vi "8chanxyplot.vi"() -> ()   [LabVIEW 2013]
doc: "Cont(inuous) Acq(uire) & Chart (hw timed) demonstrates the hardware timed, non-buffered technique of data acquisition. The scan clock on the board controls acquisition timing. Acquired scans are read directly from the device's FIFO using AI Single Scan. \n\nThe acquisition is configured with no buffer, and the on-board scan clock started at the selected scan rate. In the first loop iteration, the newest (most recent) scan is read from the FIFO. In each subsequent loop iteration AI Single Scan is called to read the oldest scan from the FIFO. Then if a scan is missed because the acquisition does not keep up, an error message will be displayed, and the acquisition stopped. Each scan is plotted on the chart after it is read. \n\nA common reason to use non-buffered acquisition is that some kind of processing needs to be done for each data point. You will probably want to add more functions to the diagram to customize this VI for your application. The acquisition rate you can achieve depends on how much processing and display the VI must do. This VI calls a subVI named My Single-Scan Processing. Add whatever processing you need to this subVI, or replace it with one of your own. The data processing subVI also demonstrates how to use error clusters in your own subVIs, so they can be included in the error data flow chain.\n\nBefore running this VI, set the values of the controls on the front panel. Select Show Help Window from the Help menu to see a description of each control. If the values you select for all the controls are values you will usually use, select Make Current Values Default from the Operate menu and save the VI. Or, you may save individual control's default values by popping up on the control, selecting Data Operations, then selecting Make Current Value Default, and saving the VI."
uses:
  <vilib>/DAQmx/read.llb/DAQmx Read (Analog 2D DBL NChan NSamp).vi
  BiaxGlobals.vi
  <vilib>/DAQmx/create/channels.llb/DAQmx Create Channel (AI-Voltage-Basic).vi
  <vilib>/DAQmx/configure/timing.llb/DAQmx Timing (Sample Clock).vi
  Homegrown2/effectiveglobals.vi
  <vilib>/DAQmx/miscellaneous.llb/DAQmx Fill In Error Info.vi
panel:
  in  "Show plot":bool
  out "Zero Voltage Y":dbl
  in  "Calibration y-axis (V/unit)":dbl=0.0119 format="%#_6f"
  in  "Select y-axis":string(combo)="Shear load"
  in  "Calibration x-axis (V/unit)":dbl=1.5233 format="%#_6f"
  in  "Select x-axis":string(combo)="LP displacement"
  out "Offset Voltage 2":dbl=-4.85
  in  "Offset DCDT 2":bool
  out "Offset Voltage 1":dbl=-4.85
  in  "Offset DCDT 1":bool
  in  "Zero y-axis":bool
  in  "Reset plot":bool
  out "Zero Voltage X":dbl
  in  "Zero X-axis":bool
  out "Shear Load vs Displacement":cluster{"Y":dbl[], "Y":dbl[]}[](graph)
  out "element 11":string
  out "element 10":string
  out "element 9":string
  out "element 8":string
  out "element 7":string
  out "element 6":string
  out "element 5":string
  out "element 4":string
  out "element 3":string
  out "element 2":string
  out "element":string
  out "element":string
  out "Stress-strain-temp vs time (Voltage)":dbl[][](graph)
  out "Array 13":i32[][](array[numeric])
  out "Array 12":i32[][](array[numeric])
  out "AUX8 (ch11)":dbl format="%.4f"
  out "AUX7 (ch10)":dbl format="%.4f"
  out "Array 11":i32[][](array[numeric])
  out "Array 10":i32[][](array[numeric])
  out "AUX6 (ch9)":dbl format="%.4f"
  out "AUX5 (ch8)":dbl format="%.4f"
  out "Array 9":i32[][](array[numeric])
  out "Array 8":i32[][](array[numeric])
  out "Array 7":i32[][](array[numeric])
  out "Array 6":i32[][](array[numeric])
  out "Array 5":i32[][](array[numeric])
  out "Array 4":i32[][](array[numeric])
  out "Array 3":i32[][](array[numeric])
  out "Array 2":i32[][](array[numeric])
  out "Array":i32[][](array[numeric])
  out "AUX4 (ch7)":dbl format="%.4f"
  out "AUX3 (ch6)":dbl format="%.4f"
  out "AUX2 (ch5)":dbl format="%.4f"
  out "AUX1 (ch4)":dbl format="%.4f"
  out "10000":bool
  in  "10 kHz":bool
  out "Processor scan rate":i32
  out "Present sample number":i32
  in  "1 Hz":bool
  out "1":bool
  out "10":bool
  out "100":bool
  out "1000":bool
  in  "10 Hz":bool
  in  "100 Hz":bool
  in  "1000 Hz":bool
  out "Data Recording Rate":i32(slide) scale=1.0..10000.0
  out "Write interval":i32
  out "Write countdown":i32
  out "Time into data acq. (s)":i32
  out "Saved sample No.":i32
  out "Record rate (samp/s)":i32
  out "No. of scans in backlog":i32
  out "Vert LVDT (ch3)":dbl format="%.4f"
  out "Vert Load (ch2)":dbl format="%.4f"
  out "Hor Load (ch0)":dbl format="%.4f"
  out "Hor LVDT (ch1)":dbl format="%.4f"
  in  "stop":bool
  # "Input Signals (volts)"
  # "To File (32 bit)"
  # "S\nI\nG\nN\nA\nL\n\nV\nO\nL\nT\nA\nG\nE"
  # "Timestamp"
  # "Acquisition Statistics"
  # "Data Recording Info"
  # "Sample (point) Number"
  # "NOTE:  This instrument will write data (time channel then Channels 0-3) to a user defined filename.  The file is written in binary format without a header.  The time channel is comprised of numbers indicating the data recording frequency (eg 1, 10, 100, 1000, 10000  samples per second)."
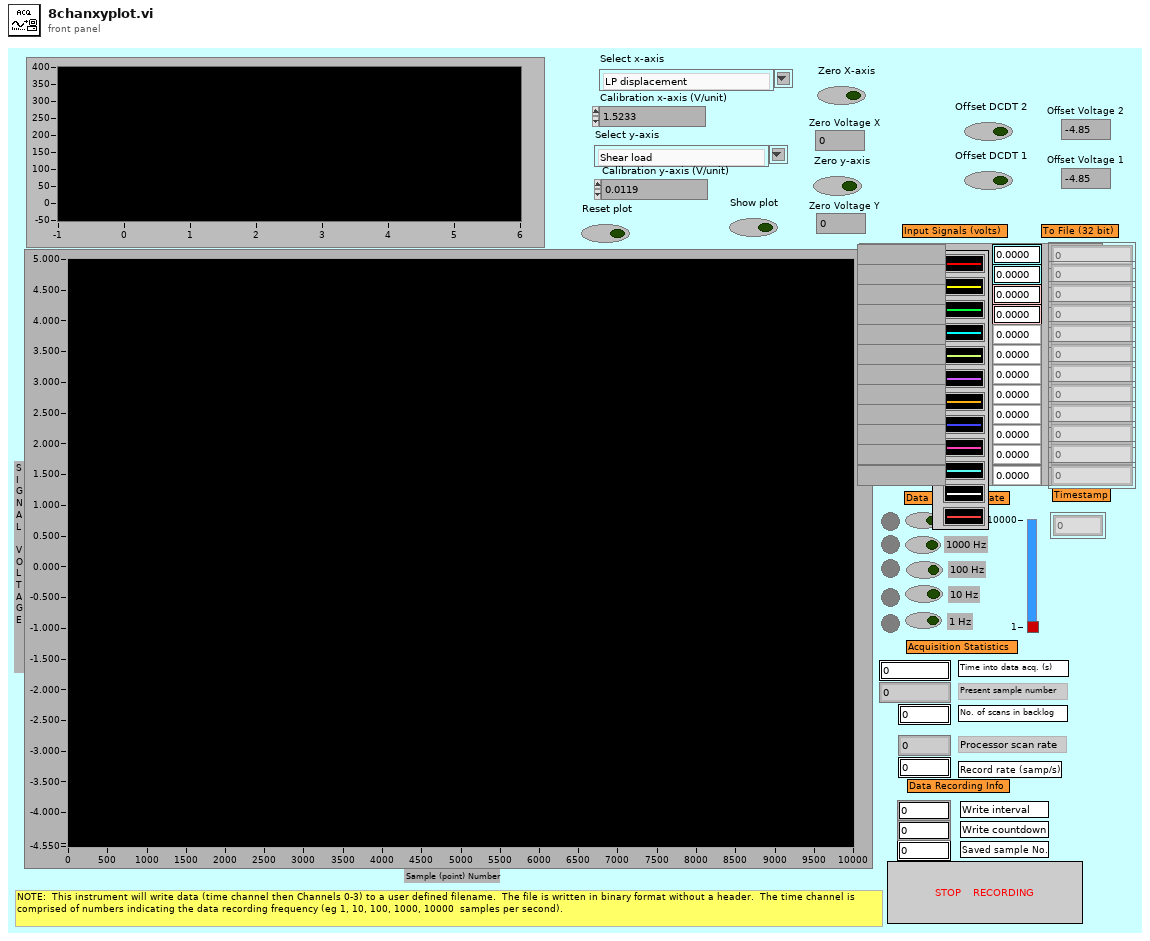
[diagram p1: front panel]
types:
  T1 = enum16{"big-endian, network order", "native, host order", "little-endian"}
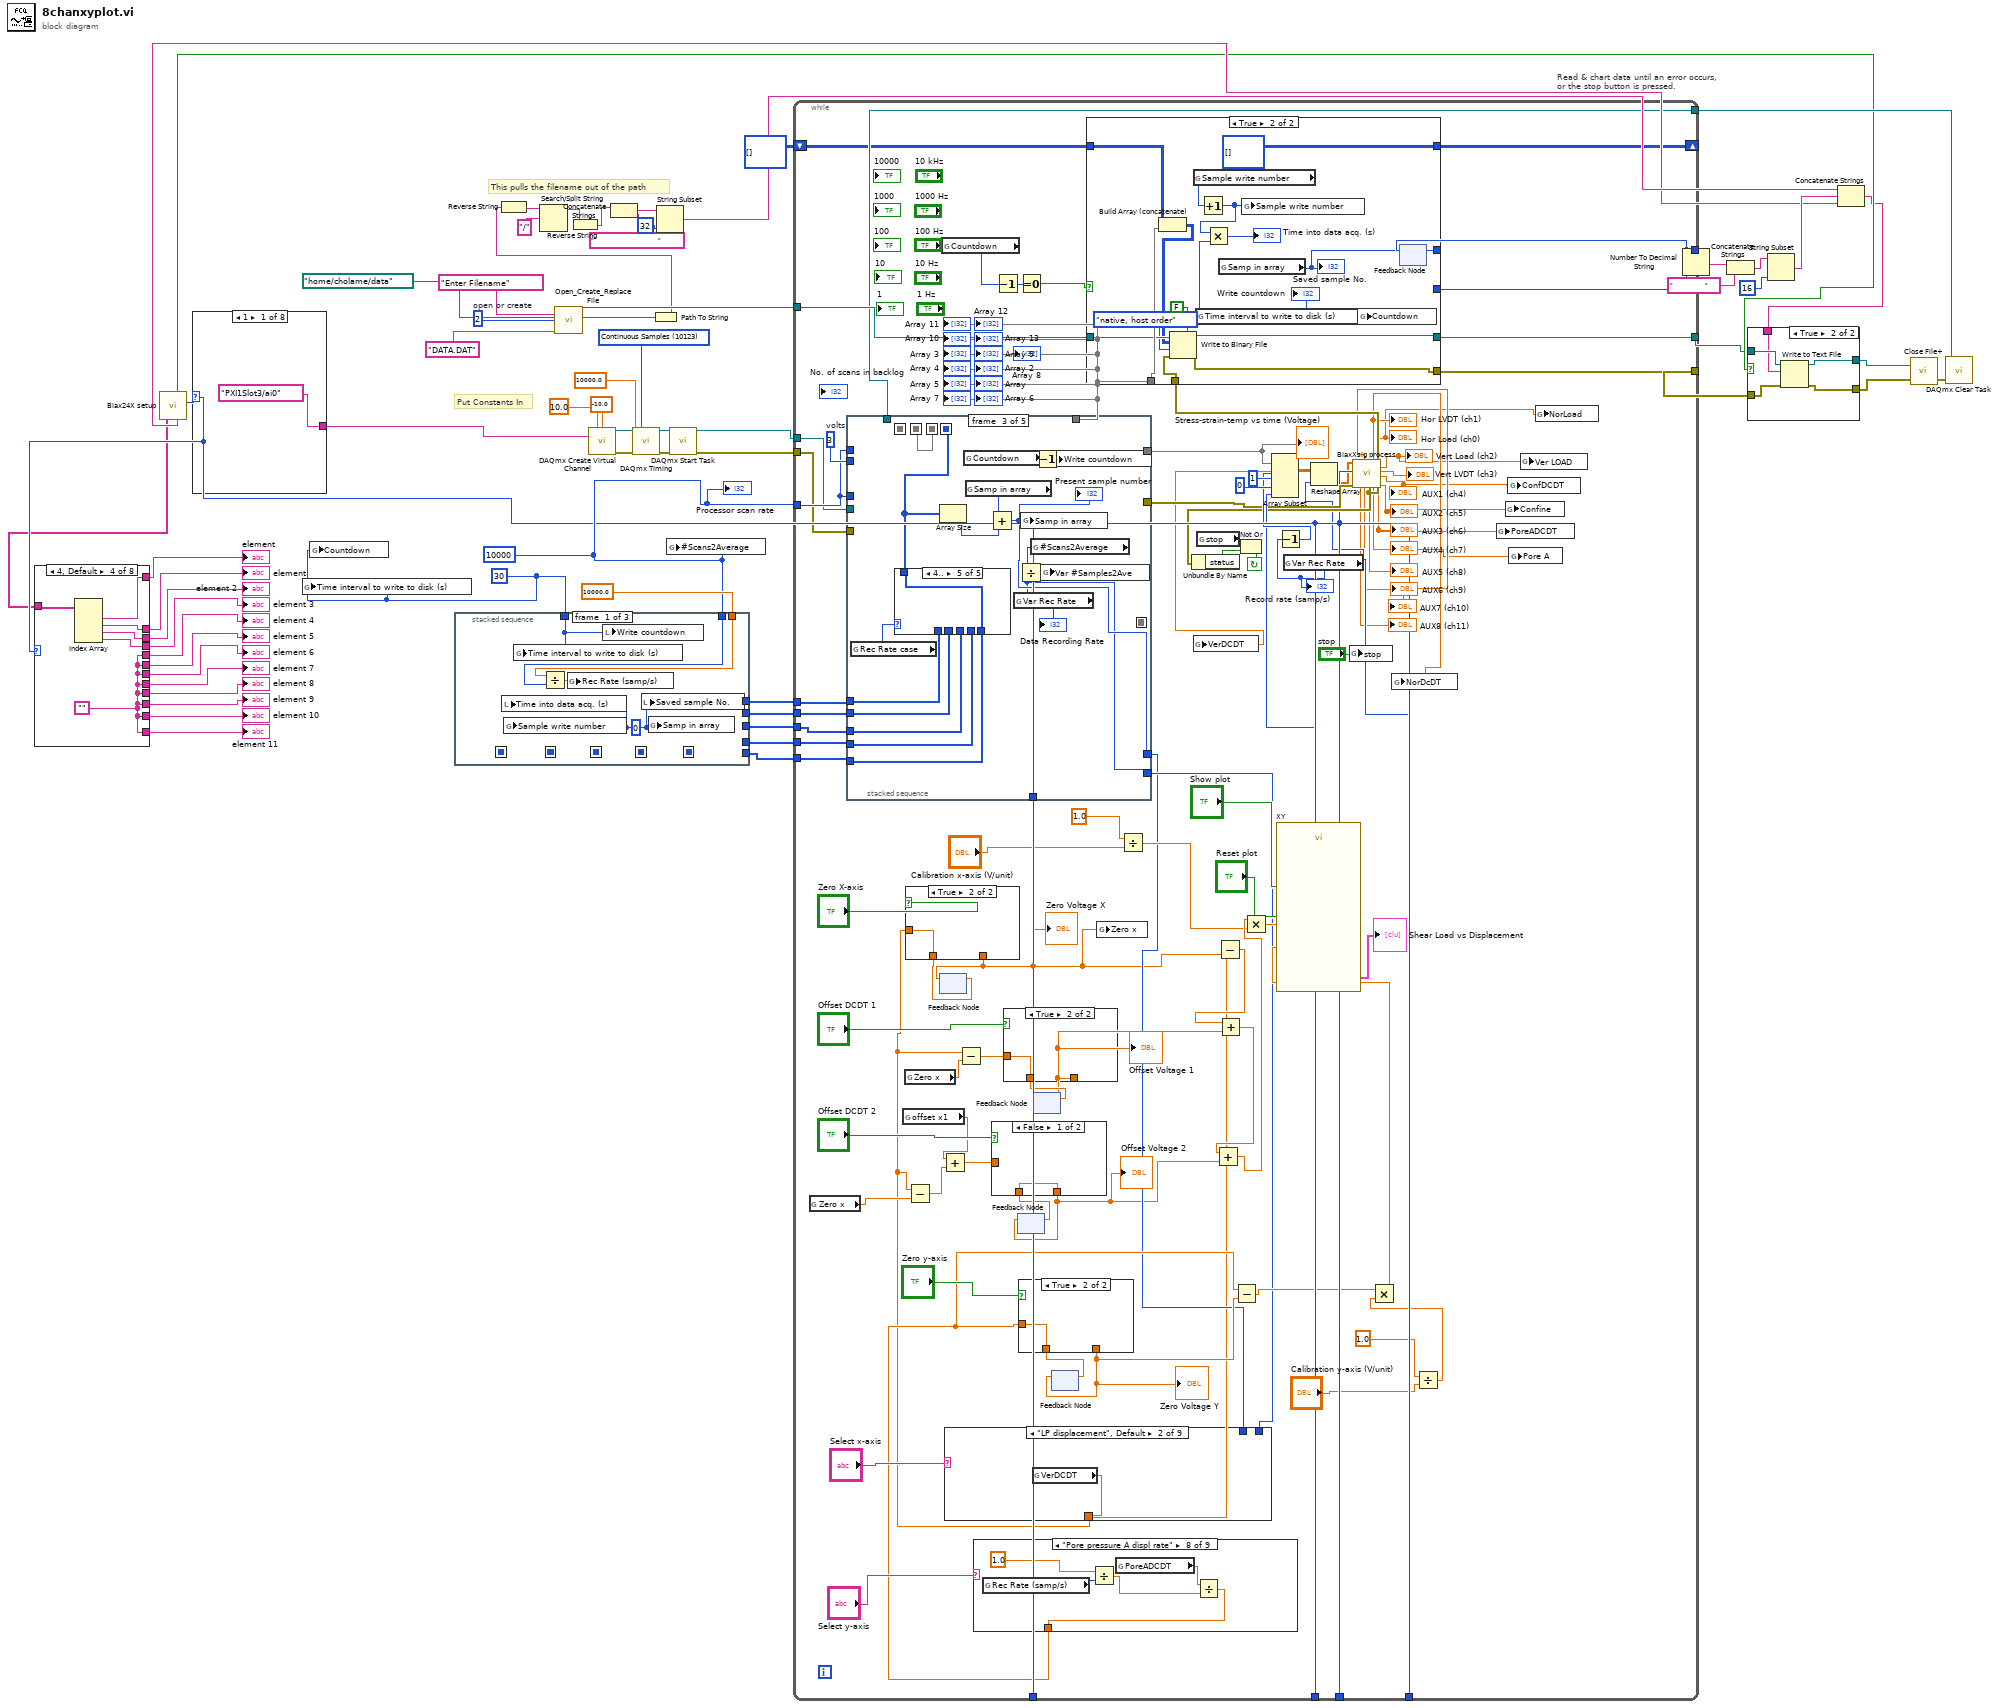
[diagram p0: block diagram]
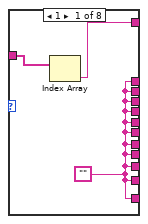
[diagram p2: hidden frame]
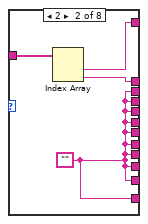
[diagram p3: hidden frame]
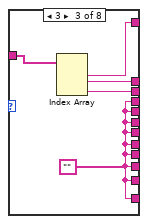
[diagram p4: hidden frame]
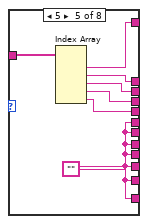
[diagram p5: hidden frame]
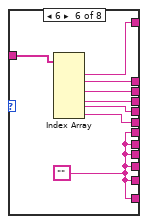
[diagram p6: hidden frame]
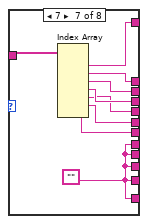
[diagram p7: hidden frame]
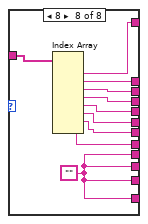
[diagram p8: hidden frame]
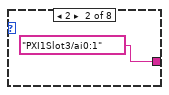
[diagram p10: hidden frame]
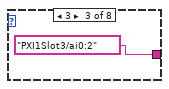
[diagram p11: hidden frame]
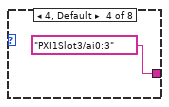
[diagram p12: hidden frame]
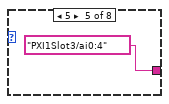
[diagram p13: hidden frame]
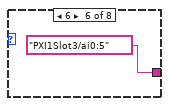
[diagram p14: hidden frame]
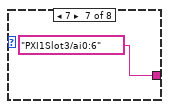
[diagram p15: hidden frame]
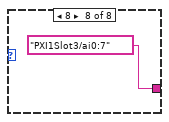
[diagram p16: hidden frame]
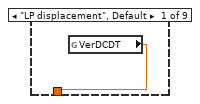
[diagram p17: hidden frame]
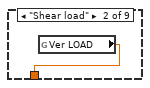
[diagram p18: hidden frame]
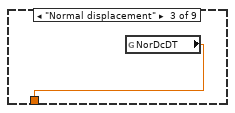
[diagram p19: hidden frame]
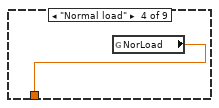
[diagram p20: hidden frame]
diagram:
  w34 = 10000 ("Number of scans")
  w33 = 30 ("Write time int (s)")
  w43 = 10123 items=["Finite Samples"=10178, "Continuous Samples"=10123, "Hardware Timed Single Point"=12522] ("sample mode")
  w64 = 2  # open or create
  # "This pulls the filename out of the path"
  # "Put Constants In"
  n1 = call "Biax24X setup.vi"() -> ("Footer String"=w22:string, "Number of Channels"=w15:i32, "ASCII footer 2"=w21:bool, "Channel Names"=w14:string[])  [unwired: 1 in, 4 out]
  n2 = case shown="4, Default" w15 {
    tunnel: w14 -> [w66 w70 w75 w81 w88 w96 w105 w116]
    tunnel: [w65 w71 w76 w82 w89 w97 w106 w115] -> w13
    tunnel: [w67 w69 w74 w80 w87 w95 w104 w114] -> w12
    tunnel: [w67 w68 w73 w79 w86 w94 w103 w113] -> w11
    tunnel: [w67 w68 w72 w78 w85 w93 w102 w112] -> w10
    tunnel: [w67 w68 w72 w77 w84 w92 w101 w111] -> w9
    tunnel: [w67 w68 w72 w77 w83 w91 w100 w110] -> w8
    tunnel: [w67 w68 w72 w77 w83 w90 w99 w109] -> w7
    tunnel: [w67 w68 w72 w77 w83 w90 w98 w108] -> w6
    tunnel: [w67 w68 w72 w77 w83 w90 w98 w107] -> w5
    tunnel: [w67 w68 w72 w77 w83 w90 w98 w107] -> w4
    tunnel: [w67 w68 w72 w77 w83 w90 w98 w107] -> w3
    tunnel: [w67 w68 w72 w77 w83 w90 w98 w107] -> w2
    frame 1 {
      w67 = ""
      n3 = Index Array(array=w66) -> (element=w65:string)  [unwired: 1 in]
    }
    frame 2 {
      w68 = ""
      n4 = Index Array(array=w70) -> (element #1=w71:string, element #2=w69:string)  [unwired: 2 in]
    }
    frame 3 {
      w72 = ""
      n5 = Index Array(array=w75) -> (element #1=w76:string, element #2=w74:string, element #3=w73:string)  [unwired: 3 in]
    }
    frame 4, Default {
      w77 = ""
      n6 = Index Array(array=w81) -> (element #1=w82:string, element #2=w80:string, element #3=w79:string, element #4=w78:string)  [unwired: 4 in]
    }
    frame 5 {
      w83 = ""
      n7 = Index Array(array=w88) -> (element #1=w89:string, element #2=w87:string, element #3=w86:string, element #4=w85:string, element #5=w84:string)  [unwired: 5 in]
    }
    frame 6 {
      w90 = ""
      n8 = Index Array(array=w96) -> (element #1=w97:string, element #2=w95:string, element #3=w94:string, element #4=w93:string, element #5=w92:string, element #6=w91:string)  [unwired: 6 in]
    }
    frame 7 {
      w98 = ""
      n9 = Index Array(array=w105) -> (element #1=w106:string, element #2=w104:string, element #3=w103:string, element #4=w102:string, element #5=w101:string, element #6=w100:string, element #7=w99:string)  [unwired: 7 in]
    }
    frame 8 {
      w107 = ""
      n10 = Index Array(array=w116) -> (element #1=w115:string, element #2=w114:string, element #3=w113:string, element #4=w112:string, element #5=w111:string, element #6=w110:string, element #7=w109:string, element #8=w108:string)  [unwired: 8 in]
    }
  }
  "element" <- w13
  "element" <- w12
  "element 2" <- w11
  "element 3" <- w10
  "element 4" <- w9
  "element 5" <- w8
  "element 6" <- w7
  "element 7" <- w6
  "element 8" <- w5
  "element 9" <- w4
  "element 10" <- w3
  "element 11" <- w2
  n11 = case shown="1" w15 {
    tunnel: [tag "PXI1Slot3/ai0" ("physical channels") tag "PXI1Slot3/ai0:1" ("physical channels") tag "PXI1Slot3/ai0:2" ("physical channels") tag "PXI1Slot3/ai0:3" ("physical channels") tag "PXI1Slot3/ai0:4" ("physical channels") tag "PXI1Slot3/ai0:5" ("physical channels") tag "PXI1Slot3/ai0:6" ("physical channels") tag "PXI1Slot3/ai0:7" ("physical channels")] -> w30
    frame 1 {
    }
    frame 2 {
    }
    frame 3 {
    }
    frame 4, Default {
    }
    frame 5 {
    }
    frame 6 {
    }
    frame 7 {
    }
    frame 8 {
    }
  }
  n12 = global write "BiaxGlobals.vi" "Time interval to write to disk (s)"(w33) -> ()
  n13 = global write "BiaxGlobals.vi" "Countdown"(w33) -> ()
  n14 = stacked-sequence {
    seq-local: [_ w145 _] -> [_ _ w158]
    seq-local: [_ w142 _] -> [_ _ w155]
    seq-local: [_ w137 _] -> [_ _ w157]
    seq-local: [_ w136 _] -> [_ _ w156]
    seq-local: [_ w131 _] -> [_ _ w154]
    tunnel: w33 -> [w125 _ _]
    tunnel: w34 -> [w129 _ _]
    tunnel: sgl 10000.0 ("actual scan rate") -> [w127 _ _]
    tunnel: [_ _ w158] -> w59
    tunnel: [_ _ w155] -> w58
    tunnel: [_ _ w157] -> w57
    tunnel: [_ _ w156] -> w56
    tunnel: [_ _ w154] -> w55
    frame #0 {
      w126 = i16 0
      n15 = local write "Time into data acq. (s)"(w126) -> ()
      n16 = global write "BiaxGlobals.vi" "Sample write number"(w126) -> ()
      n17 = global write "BiaxGlobals.vi" "Time interval to write to disk (s)"(w125) -> ()
      n18 = Divide(x=w127, y=w129) -> (x/y=w128:sgl)
      n19 = global write "BiaxGlobals.vi" "Rec Rate (samp/s)"(w128) -> ()
      n20 = local write "Write countdown"(w125) -> ()
      n21 = local write "Saved sample No."(w126) -> ()
      n22 = global write "BiaxGlobals.vi" "Samp in array"(w126) -> ()
    }
    frame #1 {
      n23 = Initialize Array(i16 1, 10000) -> (w145:i16[])
      n24 = global write "BiaxGlobals.vi" "Rec Rate case"(4) -> ()
      n25 = local write "10"(FALSE) -> ()
      n26 = local write "1"(TRUE) -> ()
      n27 = Initialize Array(i16 10, 1000) -> (w142:i16[])
      n28 = local write "1000"(FALSE) -> ()
      n29 = local write "100"(FALSE) -> ()
      n30 = global read "BiaxGlobals.vi" "Time interval to write to disk (s)"() -> (→"Write interval":i32)
      n31 = Initialize Array(i16 100, 100) -> (w137:i16[])
      n32 = local write "10000"(FALSE) -> ()
      n33 = Initialize Array(i16 1000, 10) -> (w136:i16[])
      n34 = Initialize Array(i16 10000, 1) -> (w131:i16[])
      n35 = global write "BiaxGlobals.vi" "Accum Time"(0) -> ()
      n36 = global write "BiaxGlobals.vi" "Var Rec Rate"(1) -> ()
    }
    frame #2 {
    }
  }
  n37 = call <vilib>:"Open_Create_Replace File.vi"("default name"="DATA.DAT", "prompt"="Enter Filename", "function (open:0)"=w64, "start path  (Not A Path)"=path "/home/cholame/data") -> ("new file path"=w54:path, "refnum"=w61:refnum<file>)  [unwired: 4 in, 2 out]
  n38 = call-poly <vilib>:"DAQmx Create Virtual Channel.vi"("maximum value"=10.0, "minimum value"=-10.0, "physical channels"=w30) -> ("task out"=w45:refnum<k21>, "error out"=w44:errorcluster)  [unwired: 11 in]
  n39 = call-poly <vilib>:"DAQmx Timing.vi"("task/channels in"=w45, "sample mode"=w43, "rate"=10000.0, "error in"=w44) -> ("task out"=w42:refnum<k21>, "error out"=w41:errorcluster)  [unwired: 10 in]
  n40 = Path To String(path=w54) -> (string=w51:string)
  n41 = Reverse String(1:w51) -> (0:w52:string)
  n42 = Search/Split String(string=w52, search string/char (-)="/") -> (substring before match=w50:string)  [unwired: 1 in, 2 out]
  n43 = Reverse String(1:w50) -> (0:w46:string)
  n44 = Concatenate Strings(w46, "                                ") -> (w48:string)
  n45 = String Subset(string=w48, length (rest)=32 ("length (rest)")) -> (substring=w23:string)  [unwired: 1 in]
  n46 = global write "BiaxGlobals.vi" "#Scans2Average"(w34) -> ()
  n47 = call <vilib>:"DAQmx Start Task.vi"("task/channels in"=w42, "error in"=w41) -> ("task out"=w38:refnum<k21>, "error out"=w39:errorcluster)  [unwired: 12 in]
  n48 = while "Read & chart data until an error occurs,\nor the stop button is pressed." {
    tunnel: w55 -> [w223]
    tunnel: w56 -> [w226]
    tunnel: w57 -> [w227]
    tunnel: w58 -> [w228]
    tunnel: w59 -> [w229]
    shift-left: i16[][] [] -> [w214]
    shift-right: [w244] -> _
    tunnel: w34 -> [w230]
    tunnel: [w245] -> w17
    tunnel: [w246] -> w20
    tunnel: w61 -> [w247]
    tunnel: w15 -> [w222]
    tunnel: w15 -> [w217]
    tunnel: w15 -> [w221]
    tunnel: w15 -> [w218]
    tunnel: w39 -> [w210]
    tunnel: w38 -> [w209]
    tunnel: [w238] -> w37
    tunnel: [w207] -> w29
    stop <- w243 continue-if-true
    w237 = 3  # volts
    n49 = global read "effectiveglobals.vi" "Zero x"() -> (w164:dbl)
    n50 = stacked-sequence {
      seq-local: [w280 _ _ _ _] -> [_ w289 _ _ _]
      seq-local: [_ w289 _ _ _] -> [_ _ w317 _ _]
      seq-local: [_ _ w317 _ _] -> [_ _ _ w339 _]
      seq-local: [_ _ w316 _ _] -> [_ _ _ _ w366]
      seq-local: [_ _ _ w336 _] -> [_ _ _ _ w362]
      tunnel: [w286 _ _ _ _] -> w238
      tunnel: w237 -> [_ _ _ _ _]
      tunnel: w230 -> [w282 _ _ w338 _]
      tunnel: [w285 _ _ _ _] -> w220
      tunnel: [_ _ _ _ w362] -> w234
      tunnel: w230 -> [_ _ _ _ w365]
      tunnel: w229 -> [_ _ w326 _ _]
      tunnel: w228 -> [_ _ w325 _ _]
      tunnel: w227 -> [_ _ w324 _ _]
      tunnel: w226 -> [_ _ w323 _ _]
      tunnel: [_ _ _ _ w363] -> w211
      tunnel: w223 -> [_ _ w315 _ _]
      tunnel: w221 -> [_ _ _ w334 _]
      tunnel: w210 -> [w284 _ _ _ _]
      tunnel: w209 -> [w283 _ _ _ _]
      tunnel: [_ _ w314 _ _] -> w170
      tunnel: [_ _ w313 _ _] -> w171
      frame #0 {
        n51 = call-poly <vilib>:"DAQmx Read.vi"("task/channels in"=w283, "number of samples per channel"=w282, "error in"=w284) -> ("task out"=w286:refnum<k21>, "data"=w281:dbl[][], "error out"=w285:errorcluster)  [unwired: 10 in]
        n52 = Transpose 2D Array(2D array=w281) -> (transposed array=w280:dbl[][])
      }
      frame #1 {
        n53 = local read "1000 Hz"() -> (w292:bool)
        n54 = local read "100 Hz"() -> (w291:bool)
        n55 = local read "10 Hz"() -> (w290:bool)
        n56 = local read "1 Hz"() -> (w288:bool)
        n57 = local read "10 kHz"() -> (w287:bool)
        n58 = case shown="True" w287 {
          frame False {
          }
          frame True {
            w293 = FALSE
            n59 = local write "1"(w293) -> ()
            n60 = local write "10"(w293) -> ()
            n61 = local write "100"(w293) -> ()
            n62 = local write "1000"(w293) -> ()
            n63 = local write "10000"(TRUE ("10x")) -> ()
            n64 = global write "BiaxGlobals.vi" "Rec Rate case"(0) -> ()
            n65 = global write "BiaxGlobals.vi" "Var Rec Rate"(10000) -> ()
          }
        }
        n66 = case shown="True" w292 {
          frame False {
          }
          frame True {
            w309 = FALSE
            n67 = local write "1"(w309) -> ()
            n68 = local write "10"(w309) -> ()
            n69 = local write "100"(w309) -> ()
            n70 = local write "10000"(w309) -> ()
            n71 = local write "1000"(TRUE ("10x")) -> ()
            n72 = global write "BiaxGlobals.vi" "Rec Rate case"(1) -> ()
            n73 = global write "BiaxGlobals.vi" "Var Rec Rate"(1000) -> ()
          }
        }
        n74 = case shown="True" w291 {
          frame False {
          }
          frame True {
            w305 = FALSE
            n75 = local write "1"(w305) -> ()
            n76 = local write "10"(w305) -> ()
            n77 = local write "1000"(w305) -> ()
            n78 = local write "10000"(w305) -> ()
            n79 = local write "100"(TRUE ("1x")) -> ()
            n80 = global write "BiaxGlobals.vi" "Rec Rate case"(2) -> ()
            n81 = global write "BiaxGlobals.vi" "Var Rec Rate"(100) -> ()
          }
        }
        n82 = case shown="True" w290 {
          frame False {
          }
          frame True {
            w301 = FALSE
            n83 = local write "1"(w301) -> ()
            n84 = local write "100"(w301) -> ()
            n85 = local write "1000"(w301) -> ()
            n86 = local write "10000"(w301) -> ()
            n87 = local write "10"(TRUE ("0.1x")) -> ()
            n88 = global write "BiaxGlobals.vi" "Rec Rate case"(3) -> ()
            n89 = global write "BiaxGlobals.vi" "Var Rec Rate"(10) -> ()
          }
        }
        n90 = case shown="True" w288 {
          frame False {
          }
          frame True {
            w297 = FALSE
            n91 = local write "10"(w297) -> ()
            n92 = local write "100"(w297) -> ()
            n93 = local write "1000"(w297) -> ()
            n94 = local write "10000"(w297) -> ()
            n95 = local write "1"(TRUE) -> ()
            n96 = global write "BiaxGlobals.vi" "Rec Rate case"(4) -> ()
            n97 = global write "BiaxGlobals.vi" "Var Rec Rate"(1) -> ()
          }
        }
      }
      frame #2 {
        n98 = global read "BiaxGlobals.vi" "Rec Rate case"() -> (w322:i32)
        n99 = case shown="4.." w322 {
          tunnel: w326 -> [w329 _ _ _ _]
          tunnel: [w329 w330 w331 w332 w333] -> w316
          tunnel: w325 -> [_ w330 _ _ _]
          tunnel: w324 -> [_ _ w331 _ _]
          tunnel: w323 -> [_ _ _ w332 _]
          tunnel: w315 -> [_ _ _ _ w333]
          frame ..0 {
          }
          frame 1 {
          }
          frame 2 {
          }
          frame 3 {
          }
          frame 4.. {
          }
        }
        n100 = Array Size(array=w316) -> (size(s)=w320:i32)
        n101 = global read "BiaxGlobals.vi" "Countdown"() -> (w319:i32)
        n102 = global read "BiaxGlobals.vi" "Samp in array"() -> (w321:i32)
        n103 = Add(x=w321, y=w320) -> (x+y=w314:i32)
        "Present sample number" <- w314
        n104 = global read "BiaxGlobals.vi" "Var Rec Rate"() -> (w313:i32)
        "Data Recording Rate" <- w313
        n105 = global write "BiaxGlobals.vi" "Samp in array"(w314) -> ()
        n106 = global read "BiaxGlobals.vi" "#Scans2Average"() -> (w328:i16)
        n107 = Divide(x=w328, y=w313) -> (x/y=w327:dbl)
        n108 = Decrement(x=w319) -> (x-1=w318:i32)
        n109 = global write "BiaxGlobals.vi" "Var #Samples2Ave"(w327) -> ()
        n110 = local write "Write countdown"(w318) -> ()
      }
      frame #3 {
        n111 = To Long Integer(number=w338) -> (32bit integer=w337:i32)
        n112 = global read "BiaxGlobals.vi" "Var Rec Rate"() -> (w340:i32)
        n113 = Equal?(x=w340, y=w337) -> (x = y?=w335:bool)
        n114 = case shown="False" w335 {
          tunnel: w339 -> [w344 w356]
          tunnel: [w343 w356] -> w336
          tunnel: w334 -> [w341 _]
          frame False {
            n115 = global read "BiaxGlobals.vi" "Var Rec Rate"() -> (w342:i32)
            n116 = for {
              N: w342 -> [_]
              shift-right: [w355] -> w343
              shift-left: dbl[][] [] -> [w351]
              tunnel: w344 -> [w354]
              tunnel: w341 -> [w348]
              i -> [w349]
              n117 = global read "BiaxGlobals.vi" "Var #Samples2Ave"() -> (w346:i32)
              n118 = Multiply(x=w346, y=w349) -> (x*y=w347:i32)
              n119 = Array Subset(array=w354, index (row)=w347, length (row)=w346, index (col)=i16 0, length (col)=w348) -> (w353:dbl[][])
              n120 = call "Average Signal Voltage.vi"("voltage data"=w353) -> ("average value\nper channel"=w350:dbl[])  [unwired: 2 in]
              n121 = Build Array (concatenate)(w351, w350) -> (w355:dbl[][])
            }
          }
          frame True {
          }
        }
      }
      frame #4 {
        (unwired) 1000.0
        n122 = global read "BiaxGlobals.vi" "Accum Time"() -> (w367:dbl)
        n123 = Transpose 2D Array(2D array=w362) -> (transposed array=w361:dbl[][])
        n124 = Multiply(x=838860.8, y=w361) -> (x*y=w359:dbl[][])
        n125 = To Long Integer(number=w359) -> (32bit integer=w358:i32[][])
        n126 = Add(x=w365, y=w367) -> (x+y=w357:dbl)
        n127 = Build Array (concatenate)(w366, w358) -> (w364:i32[][])
        n128 = global write "BiaxGlobals.vi" "Accum Time"(w357) -> ()
        n129 = Transpose 2D Array(2D array=w364) -> (transposed array=w363:i32[][])
      }
    }
    "Stress-strain-temp vs time (Voltage)" <- w234
    "Array" <- w211
    "Array 2" <- w211
    "Array 3" <- w211
    "Array 4" <- w211
    "Array 5" <- w211
    "Array 6" <- w211
    "Array 7" <- w211
    "Array 8" <- w211
    "Array 9" <- w211
    "Array 10" <- w211
    "Array 11" <- w211
    "Array 12" <- w211
    "Array 13" <- w211
    n130 = global read "effectiveglobals.vi" "offset x1"() -> (w165:dbl)
    n131 = global read "effectiveglobals.vi" "Zero x"() -> (w168:dbl)
    n132 = feedback #1() -> (w169:dbl)  [unwired: 1 in]
    "Zero Voltage X" <- w169
    n133 = global read "BiaxGlobals.vi" "Countdown"() -> (w225:i32)
    n134 = case shown="\"LP displacement\", Default" "Select x-axis" {
      tunnel: [w261 w264 w265 w266 w267 w268 w269 w270 w271] -> w163
      tunnel: w170 -> [w263 _ _ _ _ _ _ _ _]
      tunnel: w171 -> [w262 _ _ _ _ _ _ _ _]
      frame "Time (s)" {
        n135 = Divide(x=w263, y=w262) -> (x/y=w261:dbl)
      }
      frame "LP displacement", Default {
        n136 = global read "effectiveglobals.vi" "VerDCDT"() -> (w264:dbl)
      }
      frame "Shear load" {
        n137 = global read "effectiveglobals.vi" "Ver LOAD"() -> (w265:dbl)
      }
      frame "Normal displacement" {
        n138 = global read "effectiveglobals.vi" "NorDcDT"() -> (w266:dbl)
      }
      frame "Normal load" {
        n139 = global read "effectiveglobals.vi" "NorLoad"() -> (w267:dbl)
      }
      frame "Confining displacement" {
        n140 = global read "effectiveglobals.vi" "ConfDCDT"() -> (w268:dbl)
      }
      frame "Confining pressure" {
        n141 = global read "effectiveglobals.vi" "Confine"() -> (w269:dbl)
      }
      frame "Pore pressure A displacement" {
        n142 = global read "effectiveglobals.vi" "PoreADCDT"() -> (w270:dbl)
      }
      frame "Pore pressure A" {
        n143 = global read "effectiveglobals.vi" "Pore A"() -> (w271:dbl)
      }
    }
    n144 = case shown="True" "Zero X-axis" {
      tunnel: [w278 w279] -> w202
      tunnel: w169 -> [w278 _]
      tunnel: w163 -> [_ w279]
      frame False {
      }
      frame True {
      }
    }
    n145 = Subtract(x=w163, y=w164) -> (x-y=w162:dbl)
    n146 = feedback-in #1(w202) -> ()
    n147 = Add(x=w165, y=w162) -> (x+y=w161:dbl)
    n148 = Subtract(x=w163, y=w168) -> (x-y=w167:dbl)
    n149 = case shown="\"Pore pressure A displ rate\"" "Select y-axis" {
      tunnel: [w248 w249 w250 w251 w252 w253 w254 w255 w260] -> w183
      frame "LP displacement", Default {
        n150 = global read "effectiveglobals.vi" "VerDCDT"() -> (w248:dbl)
      }
      frame "Shear load" {
        n151 = global read "effectiveglobals.vi" "Ver LOAD"() -> (w249:dbl)
      }
      frame "Normal displacement" {
        n152 = global read "effectiveglobals.vi" "NorDcDT"() -> (w250:dbl)
      }
      frame "Normal load" {
        n153 = global read "effectiveglobals.vi" "NorLoad"() -> (w251:dbl)
      }
      frame "Confining displacement" {
        n154 = global read "effectiveglobals.vi" "ConfDCDT"() -> (w252:dbl)
      }
      frame "Confining pressure" {
        n155 = global read "effectiveglobals.vi" "Confine"() -> (w253:dbl)
      }
      frame "Pore pressure A displacement" {
        n156 = global read "effectiveglobals.vi" "PoreADCDT"() -> (w254:dbl)
      }
      frame "Pore pressure A displ rate" {
        n157 = global read "BiaxGlobals.vi" "Rec Rate (samp/s)"() -> (w258:i32)
        n158 = Divide(x=1.0, y=w258) -> (x/y=w256:dbl)
        n159 = global read "effectiveglobals.vi" "PoreADCDT"() -> (w257:dbl)
        n160 = Divide(x=w257, y=w256) -> (x/y=w255:dbl)
      }
      frame "Pore pressure A" {
        n161 = global read "effectiveglobals.vi" "Pore A"() -> (w260:dbl)
      }
    }
    n162 = Decrement(x=w225) -> (x-1=w224:i32)
    n163 = feedback #2() -> (w159:dbl)  [unwired: 1 in]
    "Offset Voltage 2" <- w159
    n164 = case shown="False" "Offset DCDT 2" {
      tunnel: w161 -> [_ w273]
      tunnel: [w272 w273] -> w160
      tunnel: w159 -> [w272 _]
      frame False {
      }
      frame True {
      }
    }
    n165 = feedback-in #2(w160) -> ()
    n166 = Equal To 0?(x=w224) -> (x = 0?=w239:bool)
    n167 = feedback #3() -> (w166:dbl)  [unwired: 1 in]
    "Offset Voltage 1" <- w166
    n168 = case shown="True" "Offset DCDT 1" {
      tunnel: [w274 w275] -> w194
      tunnel: w166 -> [w274 _]
      tunnel: w167 -> [_ w275]
      frame False {
      }
      frame True {
      }
    }
    n169 = feedback-in #3(w194) -> ()
    n170 = feedback #4() -> (w179:dbl)  [unwired: 1 in]
    "Zero Voltage Y" <- w179
    n171 = case shown="True" "Zero y-axis" {
      tunnel: [w276 w277] -> w198
      tunnel: w179 -> [w276 _]
      tunnel: w183 -> [_ w277]
      frame False {
      }
      frame True {
      }
    }
    n172 = feedback-in #4(w198) -> ()
    n173 = global write "effectiveglobals.vi" "Zero x"(w169) -> ()
    n174 = Divide(x=1.0, y="Calibration x-axis (V/unit)") -> (x/y=w185:dbl)
    n175 = global read "BiaxGlobals.vi" "stop"() -> (w240:bool)
    n176 = Subtract(x=w163, y=w169) -> (x-y=w193:dbl)
    n177 = Add(x=w193, y=w166) -> (x+y=w190:dbl)
    n178 = Add(x=w190, y=w159) -> (x+y=w189:dbl)
    n179 = Subtract(x=w183, y=w179) -> (x-y=w197:dbl)
    n180 = Multiply(x=w189, y=w185) -> (x*y=w204:dbl)
    n181 = global read "BiaxGlobals.vi" "Var Rec Rate"() -> (w232:i32)
    "Record rate (samp/s)" <- w232
    n182 = Decrement(x=w232) -> (x-1=w231:i32)
    n183 = Array Subset(array=w234, index (row)=w231, length (row)=1, index (col)=0, length (col)=w222) -> (w235:dbl[][])
    n184 = Reshape Array(w235, w217) -> (w206:dbl[])
    n185 = global write "BiaxGlobals.vi" "stop"("stop") -> ()
    n186 = call "BiaxXsig process.vi"("voltage data"=w206, "Numeric"=w218, "error in (no error)"=w220) -> ("AUX8"=→"AUX8 (ch11)":dbl, "AUX7"=→"AUX7 (ch10)":dbl, "AUX6"=→"AUX6 (ch9)":dbl, "AUX5"=→"AUX5 (ch8)":dbl, "error out"=w219:errorcluster, "Hor LVDT"=w196:dbl, "AUX4"=w173:dbl, "Hor Load"=w178:dbl, "Vert Load"=w177:dbl, "Vert LVDT"=w203:dbl, "AUX1"=w176:dbl, "AUX2"=w175:dbl, "AUX3"=w174:dbl)  [unwired: 3 in, 1 out]
    "Hor LVDT (ch1)" <- w196
    "Hor Load (ch0)" <- w178
    "Vert Load (ch2)" <- w177
    "Vert LVDT (ch3)" <- w203
    "AUX1 (ch4)" <- w176
    "AUX2 (ch5)" <- w175
    "AUX3 (ch6)" <- w174
    "AUX4 (ch7)" <- w173
    n187 = Unbundle By Name(w219) -> ("status"=w242:bool)
    n188 = global write "effectiveglobals.vi" "VerDCDT"(w203) -> ()
    n189 = Not Or(1:w242, 2:w240) -> (0:w243:bool)
    n190 = global write "effectiveglobals.vi" "NorDcDT"(w196) -> ()
    n191 = feedback #5() -> (w207:i32)  [unwired: 1 in]
    n192 = case shown="True" w239 {
      tunnel: w211 -> [w375 w385]
      tunnel: w214 -> [w374 w386]
      tunnel: w247 -> [w373 w382]
      tunnel: [w373 w381] -> w246
      tunnel: w219 -> [w372 w383]
      tunnel: [w372 w380] -> w245
      tunnel: [w369 i16[][] []] -> w244
      tunnel: [w368 w377] -> w208
      tunnel: w207 -> [w368 _]
      frame False {
        n193 = Build Array (concatenate)(w374, w375) -> (w369:i32[][])
        n194 = global read "BiaxGlobals.vi" "Countdown"() -> (w371:i32)
        n195 = Decrement(x=w371) -> (x-1=w370:i32)
        n196 = global write "BiaxGlobals.vi" "Countdown"(w370) -> ()
      }
      frame True {
        n197 = Build Array (concatenate)(w386, w385) -> (w379:i32[][])
        n198 = Write to Binary File(file (use dialog)=w382, data=w379, error in=w383, 5:FALSE ("prepend array or string size? (T)"), 9:T1."native, host order" ("byte order (0:big-endian, network order)")) -> (refnum out=w381:refnum<file>, error out=w380:errorcluster)  [unwired: 1 in, 1 out]
        n199 = global read "BiaxGlobals.vi" "Sample write number"() -> (w390:i16)
        n200 = global read "BiaxGlobals.vi" "Time interval to write to disk (s)"() -> (w387:i32)
        "Write countdown" <- w387
        n201 = Increment(x=w390) -> (x+1=w384:i16)
        n202 = Multiply(x=w384, y=w387) -> (x*y=→"Time into data acq. (s)":i32)
        n203 = global read "BiaxGlobals.vi" "Samp in array"() -> (w377:i32)
        "Saved sample No." <- w377
        n204 = global write "BiaxGlobals.vi" "Sample write number"(w384) -> ()
        n205 = global write "BiaxGlobals.vi" "Countdown"(w387) -> ()
      }
    }
    n206 = feedback-in #5(w208) -> ()
    n207 = Divide(x=1.0, y="Calibration y-axis (V/unit)") -> (x/y=w180:dbl)
    n208 = Multiply(x=w197, y=w180) -> (x*y=w195:dbl)
    n209 = call "XY.vi"("Enable"="Show plot", "Reset"="Reset plot", "Y Input"=w195, "X Input"=w204) -> ("XY Graph"=→"Shear Load vs Displacement":cluster{"Y":dbl[], "Y":dbl[]}[])  [unwired: 6 in, 1 out]
    n210 = global write "effectiveglobals.vi" "PoreADCDT"(w174) -> ()
    n211 = global write "effectiveglobals.vi" "Confine"(w175) -> ()
    n212 = global write "effectiveglobals.vi" "ConfDCDT"(w176) -> ()
    n213 = global write "effectiveglobals.vi" "Pore A"(w173) -> ()
    n214 = global write "effectiveglobals.vi" "Ver LOAD"(w177) -> ()
    n215 = global write "effectiveglobals.vi" "NorLoad"(w178) -> ()
  }
  n216 = Number To Decimal String(number=w29) -> (decimal integer string=w28:string)  [unwired: 1 in]
  n217 = Concatenate Strings(w28, "                " ("string")) -> (w26:string)
  n218 = String Subset(string=w26, length (rest)=16 ("length (rest)")) -> (substring=w24:string)  [unwired: 1 in]
  n219 = Concatenate Strings(w23, w24, w22) -> (w16:string)
  n220 = case shown="True" w21 {
    tunnel: [w392 w396] -> w19
    tunnel: w20 -> [w392 w397]
    tunnel: w17 -> [w391 w394]
    tunnel: [w391 w395] -> w18
    tunnel: w16 -> [_ w393]
    frame False {
    }
    frame True {
      n221 = Write to Text File(file (use dialog)=w397, text=w393, error in=w394) -> (refnum out=w396:refnum<file>, error out=w395:errorcluster)  [unwired: 1 in, 1 out]
    }
  }
  n222 = call <vilib>:"Close File+.vi"("error in (no error)"=w18, "refnum"=w19) -> ("error out"=w40:errorcluster)  [unwired: 3 in, 2 out]
  n223 = call <vilib>:"DAQmx Clear Task.vi"("task in"=w37, "error in"=w40) -> ()  [unwired: 13 in, 1 out]
  "Processor scan rate" <- w34
